vi "Main.vi"() -> ()   [LabVIEW 2013]
uses:
  <vilib>/Utility/miscctls.llb/LVPointDoubleTypeDef.ctl
  <vilib>/Analysis/1siggen.llb/Ramp Pattern by Samples.vi
  <vilib>/DAQmx/create/channels.llb/DAQmx Create Channel (AO-Voltage-Basic).vi
  <vilib>/Utility/file.llb/Write To Spreadsheet File (DBL).vi
  <vilib>/Analysis/NI_AALBase.lvlib
panel:
  out "Events A":i32
  out "Events B":i32
  in  "Tab Control":enum32{"Scan", "Correlations", "Setup"}(tab)
  in  "Init":bool
  in  "Release":bool
  in  "Save":bool
  in  "Goto Cursor":bool
  in  "Select":bool
  in  "Goto Zero":bool
  in  "Start Scan":bool
  out "Scanning":bool
  in  "dt (in tc)":u32
  out "Estimated Time (ms)":dbl
  in  "Dim1Scan":cluster{"Start":dbl, "Stop":dbl, "Steps":u32}={"Start"=0.0, "Stop"=0.0, "Steps"=1} {"Steps" min=1}
  in  "Dim1":u16(ring) items=["X", "Y", "Z"]
  in  "Dim2Scan":cluster{"Start":dbl, "Stop":dbl, "Steps":u32} {"Steps" min=1}
  in  "Dim2":u16(ring) items=["Y", "Z", "none"]
  in  "Dim3Scan":cluster{"Start":dbl, "Stop":dbl, "Steps":u32} {"Steps" min=1}
  in  "Dim3":u16(ring) items=["Z", "none"]
  out "XY Graph":T1(graph)
  out "Intensity Graph":dbl[][](graph)
  in  "3rd Dim":u32
  in  "2nd Dim":u32
  out "Cursor.Cursor Position":T2
  out "XY Graph 2":cluster{"Ramp Pattern":dbl[], "Data":i32[]}(graph)
  in  "Acquire":bool
  in  "Bin Size (ps)":i32
  in  "Bin Count":i32
  out "Voltage out":dbl[](array[numeric])
  in  "Relative Position":cluster{"X":dbl, "Y":dbl, "Z":dbl} {"Z" step=1.0; "Y" step=1.0; "X" step=1.0}
  in  "Voltage Step":cluster{"X":dbl, "Y":dbl, "Z":dbl}
  in  "Center Voltage":cluster{"X":dbl, "Y":dbl, "Z":dbl}
  in  "Define as center":bool
  out "Error":errorcluster
  in  "N":u32
  in  "Device ID":i32
  in  "Channel A":i32
  in  "Channel B":i32
  out "Time Base (ps)":dbl
  out "History Graph":cluster{dbl[], dbl[]}(graph)
  out "Value":dbl
  in  "tc (ms)":u32
  in  "stop":bool
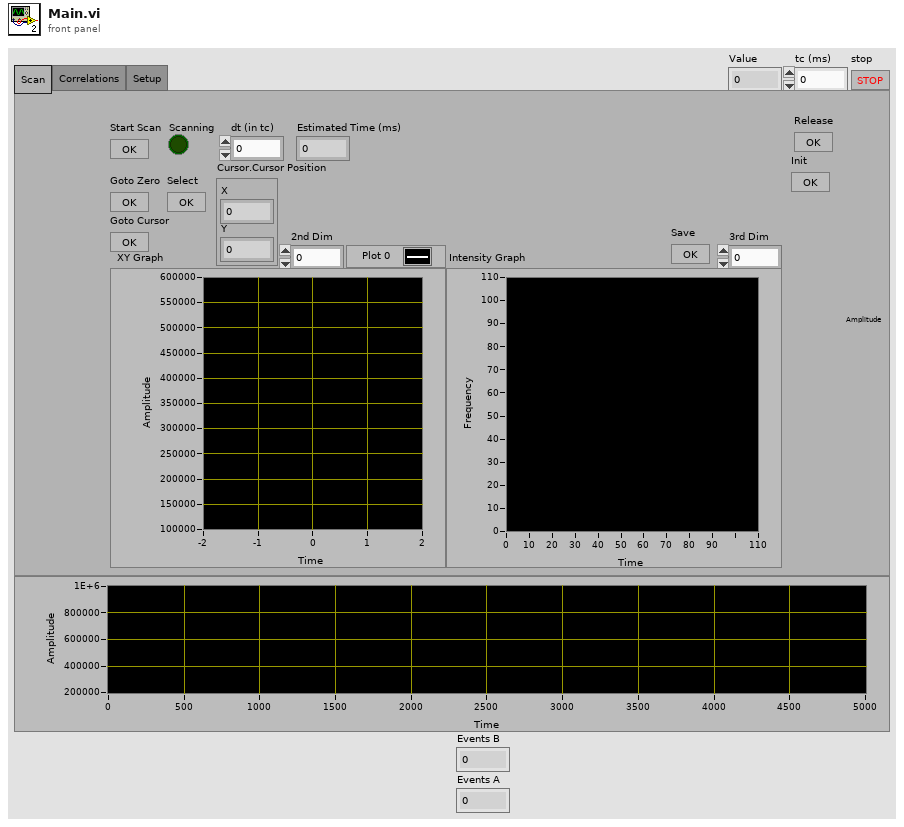
[diagram p1: front panel]
types:
  T1 = cluster{"Ramp Pattern":dbl[], "Ramp Pattern":dbl[]}
  T2 = typedef "LVPointDoubleTypeDef.ctl" = cluster{"X":dbl, "Y":dbl}
  T3 = cluster{"Voltage out[0]":dbl, "Voltage out[1]":dbl, "Voltage out[2]":dbl}
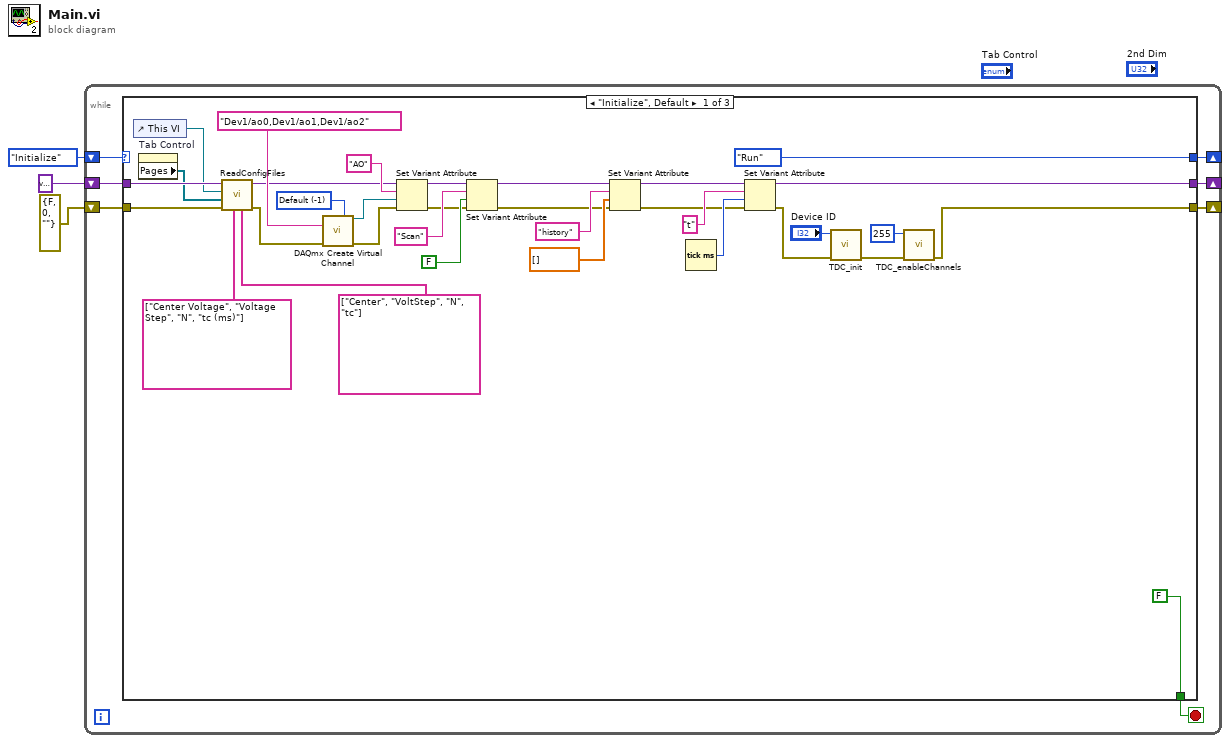
[diagram p0: block diagram]
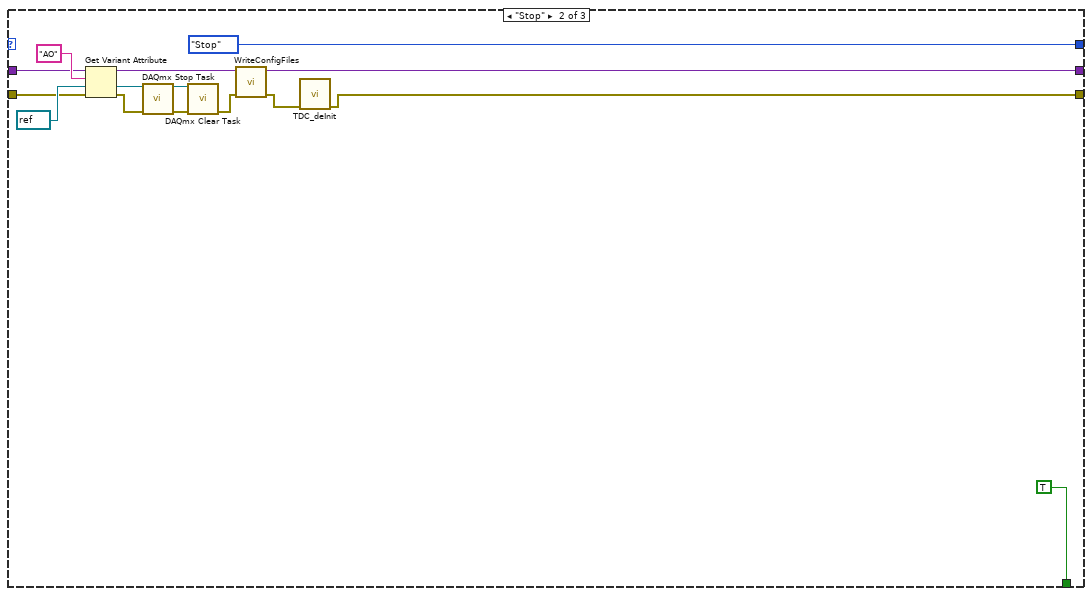
[diagram p2: hidden frame]
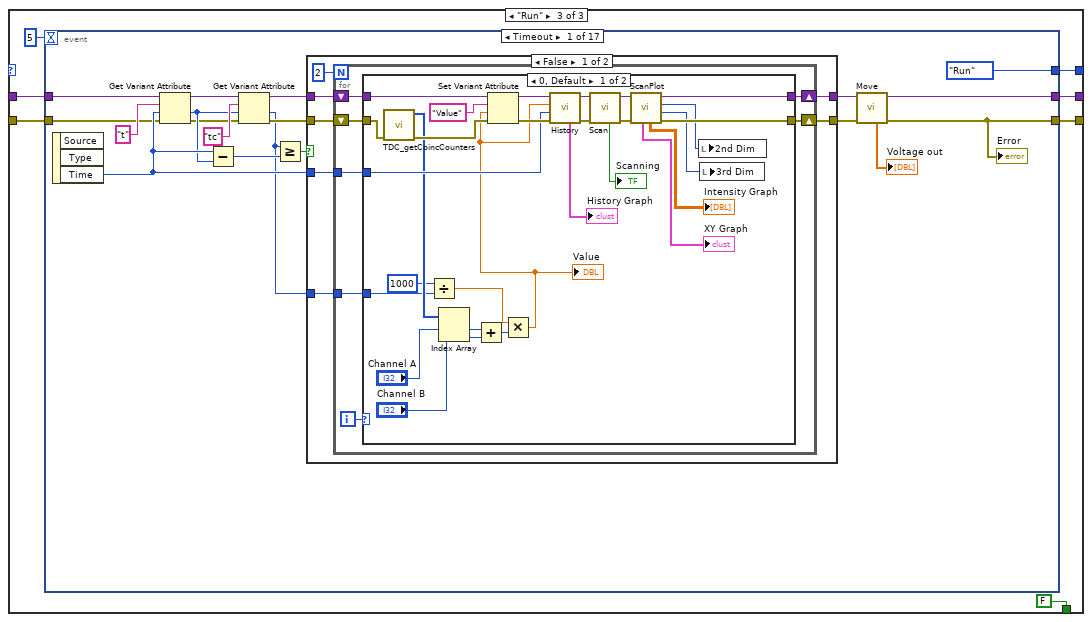
[diagram p3: hidden frame]
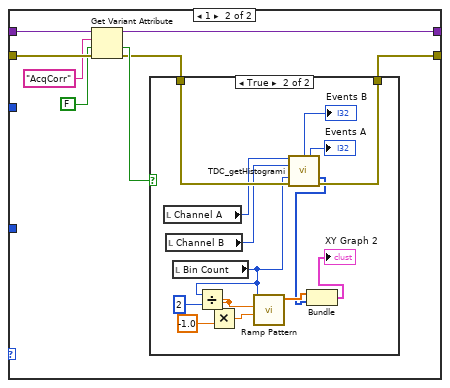
[diagram p4: hidden frame]
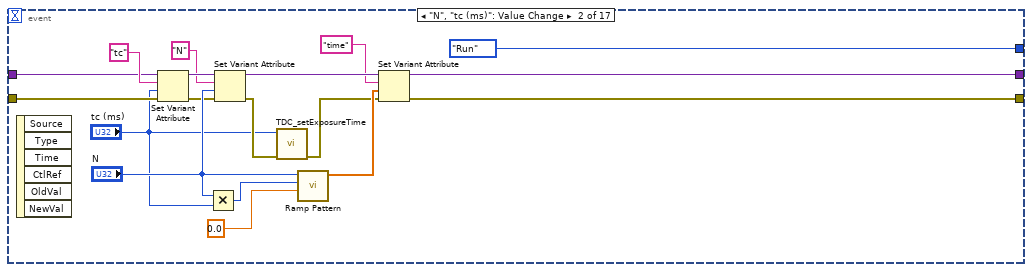
[diagram p7: hidden frame]
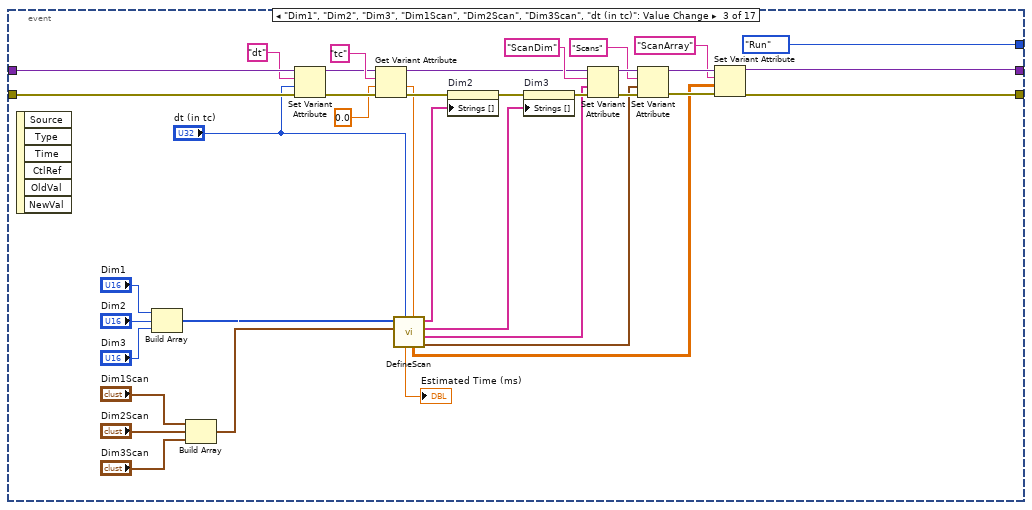
[diagram p8: hidden frame]
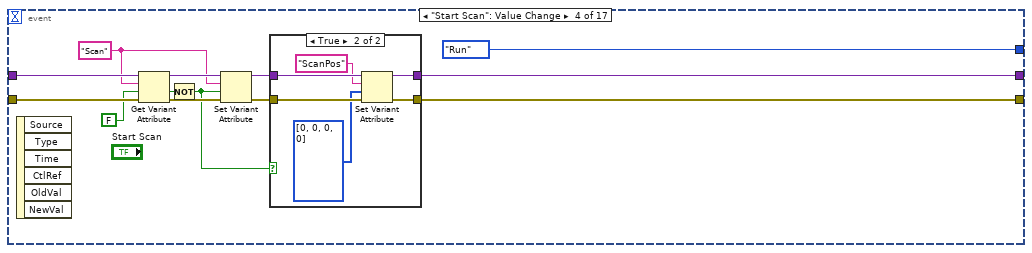
[diagram p9: hidden frame]
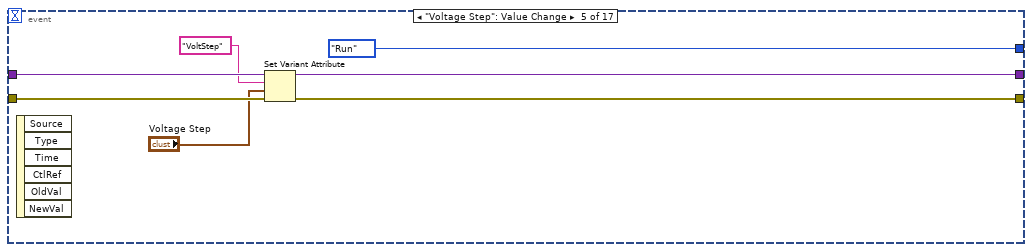
[diagram p11: hidden frame]
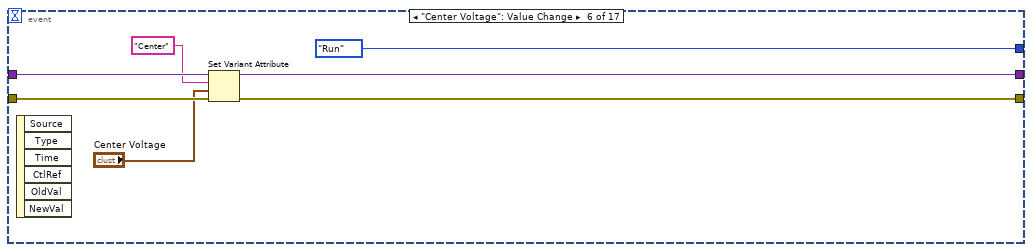
[diagram p12: hidden frame]
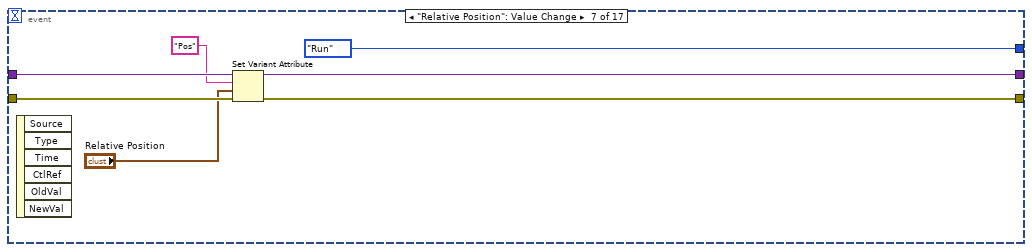
[diagram p13: hidden frame]
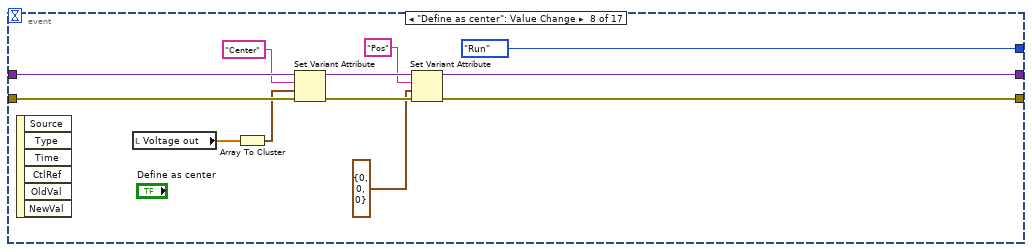
[diagram p14: hidden frame]
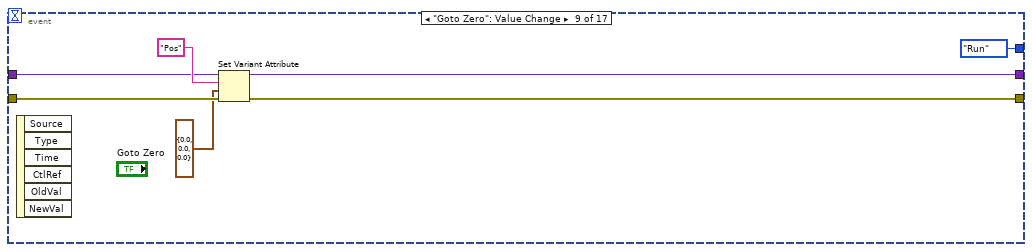
[diagram p15: hidden frame]
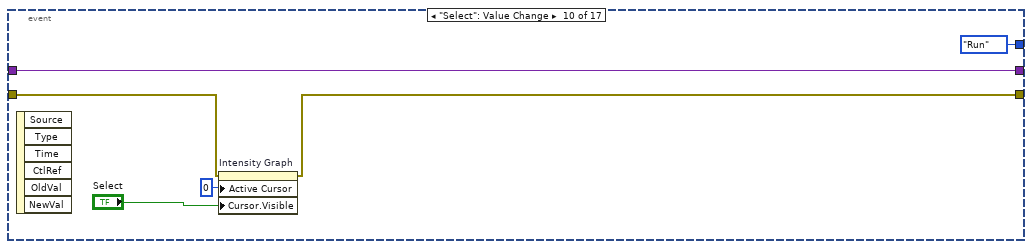
[diagram p16: hidden frame]
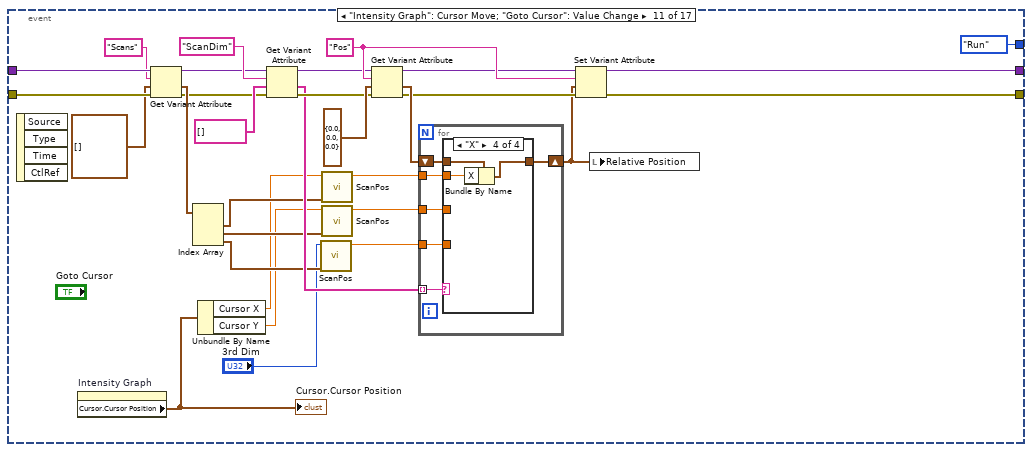
[diagram p17: hidden frame]
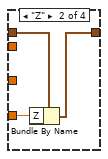
[diagram p19: hidden frame]
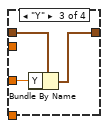
[diagram p20: hidden frame]
diagram:
  n1 = while {
    shift-right: [w9] -> _
    shift-left: enum16{"Initialize", "Run", "Stop"}."Initialize" -> [w10]
    shift-right: [w5] -> _
    shift-left: variant ("variant") -> [w7]
    shift-right: [w4] -> _
    shift-left: errorcluster {"status"=FALSE, "code"=0, "source"=""} ("error constant") -> [w6]
    stop <- w8 stop-if-true
    n2 = case shown="\"Initialize\", Default" w10 {
      tunnel: [enum16{"Initialize", "Run", "Stop"}."Run" enum16{"Initialize", "Run", "Stop"}."Stop" w65] -> w9
      tunnel: [FALSE TRUE FALSE] -> w8
      tunnel: w7 -> [w22 w54 w62]
      tunnel: w6 -> [w23 w53 w61]
      tunnel: [w35 w46 w60] -> w5
      tunnel: [w17 w44 w59] -> w4
      frame "Initialize", Default {
        w24 = -1 items=["Default"=-1, "RSE"=10083, "Differential"=10106, "Pseudodifferential"=12529] ("output terminal configuration")
        n3 = control-ref of="This VI"() -> (w14:refnum<vi>)
        n4 = property on="Tab Control" class="TabCtl (strict)"() -> ("Pages"=w13:refnum<vi>[])  [unwired: 2 in, 2 out]
        n5 = call "ReadConfigFiles.vi"("Variable"=string[] ["Center", "VoltStep", "N", "tc"], "Control"=string[] ["Center Voltage", "Voltage Step", "N", "tc (ms)"], "error in"=w23, "Pages"=w13, "reference"=w14, "variant in"=w22) -> ("error out"=w20:errorcluster, "variant out"=w21:variant)  [unwired: 4 in]
        n6 = call-poly <vilib>:"DAQmx Create Virtual Channel.vi"("output terminal configuration"=w24, "physical channels"=tag "Dev1/ao0,Dev1/ao1,Dev1/ao2", "error in"=w20) -> ("task out"=w28:refnum<k21>, "error out"=w29:errorcluster)  [unwired: 11 in]
        n7 = Set Variant Attribute(Variant=w21, name="AO", value=w28, error in=w29) -> (Variant out=w26:variant, error out=w25:errorcluster)  [unwired: 1 out]
        n8 = Set Variant Attribute(Variant=w26, name="Scan", value=FALSE, error in=w25) -> (Variant out=w34:variant, error out=w33:errorcluster)  [unwired: 1 out]
        n9 = Set Variant Attribute(Variant=w34, name="history", value=dbl[] [], error in=w33) -> (Variant out=w39:variant, error out=w36:errorcluster)  [unwired: 1 out]
        n10 = Tick Count (ms)() -> (millisecond timer value=w40:u32)
        n11 = Set Variant Attribute(Variant=w39, name="t", value=w40, error in=w36) -> (Variant out=w35:variant, error out=w19:errorcluster)  [unwired: 1 out]
        n12 = call "TDC_init.vi"("Error In"=w19, "Device ID"="Device ID") -> ("Error Out"=w18:errorcluster)  [unwired: 9 in]
        n13 = call "TDC_enableChannels.vi"("Error In"=w18, "channelMask"=255) -> ("Error Out"=w17:errorcluster)  [unwired: 9 in]
      }
      frame "Stop" {
        n14 = Get Variant Attribute(Variant=w54, name="AO", default value (empty Variant)=refnum<k21> refnum ("task out"), error in=w53) -> (duplicate Variant=w48:variant, value=w49:refnum<k21>, error out=w50:errorcluster)  [unwired: 1 out]
        n15 = call <vilib>:"DAQmx Stop Task.vi"("task/channels in"=w49, "error in"=w50) -> ("task out"=w52:refnum<k21>, "error out"=w51:errorcluster)  [unwired: 12 in]
        n16 = call <vilib>:"DAQmx Clear Task.vi"("task in"=w52, "error in"=w51) -> ("error out"=w47:errorcluster)  [unwired: 13 in]
        n17 = call "WriteConfigFiles.vi"("error in"=w47, "variant in"=w48) -> ("error out"=w45:errorcluster, "variant out"=w46:variant)  [unwired: 8 in]
        n18 = call "TDC_deInit.vi"("Error In"=w45) -> ("Error Out"=w44:errorcluster)  [unwired: 10 in]
      }
      frame "Run" {
        n19 = event shown="[0] Timeout" {
          selector: _ -> [_ _ _ _ _ _ _ _ _ _ _ _ _ _ _ _ _]
          dyn-events: _ -> [_ _ _ _ _ _ _ _ _ _ _ _ _ _ _ _ _]
          timeout: 5 -> [_ _ _ _ _ _ _ _ _ _ _ _ _ _ _ _ _]
          tunnel: [enum16{"Initialize", "Run", "Stop"}."Run" enum16{"Initialize", "Run", "Stop"}."Run" enum16{"Initialize", "Run", "Stop"}."Run" enum16{"Initialize", "Run", "Stop"}."Run" enum16{"Initialize", "Run", "Stop"}."Run" enum16{"Initialize", "Run", "Stop"}."Run" enum16{"Initialize", "Run", "Stop"}."Run" enum16{"Initialize", "Run", "Stop"}."Run" enum16{"Initialize", "Run", "Stop"}."Run" enum16{"Initialize", "Run", "Stop"}."Run" enum16{"Initialize", "Run", "Stop"}."Run" enum16{"Initialize", "Run", "Stop"}."Run" enum16{"Initialize", "Run", "Stop"}."Run" enum16{"Initialize", "Run", "Stop"}."Run" enum16{"Initialize", "Run", "Stop"}."Run" enum16{"Initialize", "Run", "Stop"}."Stop" enum16{"Initialize", "Run", "Stop"}."Stop"] -> w65
          tunnel: w62 -> [w73 w156 w202 w216 w231 w238 w245 w257 w263 w271 w301 w335 w348 w357 w370 w373 w380]
          tunnel: w61 -> [w72 w155 w201 w215 w230 w237 w244 w255 w262 w267 w300 w332 w347 w356 w369 w372 w377]
          tunnel: [w68 w154 w186 w206 w229 w236 w243 w254 w261 w271 w274 w335 w346 w355 w370 w373 w380] -> w60
          tunnel: [w67 w153 w185 w205 w228 w235 w242 w253 w260 w266 w273 w333 w342 w354 w369 w371 w376] -> w59
          event Timeout {
            n20 = event-data() -> ("Time"=w78:u32)  [unwired: 1 in, 2 out]
            n21 = Get Variant Attribute(Variant=w73, name="t", default value (empty Variant)=w78, error in=w72) -> (duplicate Variant=w77:variant, value=w75:u32, error out=w74:errorcluster)  [unwired: 1 out]
            n22 = Subtract(x=w78, y=w75) -> (x-y=w80:u32)
            n23 = Get Variant Attribute(Variant=w77, name="tc", default value (empty Variant)=w75, error in=w74) -> (duplicate Variant=w71:variant, value=w66:u32, error out=w70:errorcluster)  [unwired: 1 out]
            n24 = Greater Or Equal?(x=w66, y=w80) -> (x >= y?=w79:bool)
            n25 = case shown="False" w79 {
              tunnel: w78 -> [w88 _]
              tunnel: w71 -> [w89 w149]
              tunnel: w70 -> [w85 w148]
              tunnel: [w87 w149] -> w68
              tunnel: [w86 w148] -> w67
              tunnel: w66 -> [w84 _]
              frame False {
                n26 = for {
                  N: 2 -> [_]
                  tunnel: w88 -> [w95]
                  tunnel: w84 -> [w91]
                  shift-right: [w94] -> w87
                  shift-left: w89 -> [w96]
                  shift-right: [w93] -> w86
                  shift-left: w85 -> [w92]
                  i -> [w90]
                  n27 = case shown="0, Default" w90 {
                    tunnel: w96 -> [w124 w132]
                    tunnel: w95 -> [w119 _]
                    tunnel: [w114 w130] -> w94
                    tunnel: [w113 w125] -> w93
                    tunnel: w92 -> [w108 w131]
                    tunnel: w91 -> [w100 _]
                    frame 0, Default {
                      n28 = call "TDC_getCoincCounters.vi"("Error In"=w108) -> ("Error Out"=w107:errorcluster, "Coincidence Counters"=w106:i32[])  [unwired: 9 in]
                      n29 = Divide(x=1000, y=w100) -> (x/y=w98:dbl)
                      n30 = Index Array(array=w106, index #1="Channel A", index #2="Channel B") -> (element #1=w102:i32, element #2=w103:i32)
                      n31 = Add(x=w102, y=w103) -> (x+y=w99:i32)
                      n32 = Multiply(x=w98, y=w99) -> (x*y=w97:dbl)
                      "Value" <- w97
                      n33 = Set Variant Attribute(Variant=w124, name="Value", value=w97, error in=w107) -> (Variant out=w121:variant, error out=w122:errorcluster)  [unwired: 1 out]
                      n34 = call "History.vi"("error in"=w122, "time"=w119, "Value"=w97, "variant in"=w121) -> ("error out"=w117:errorcluster, "variant out"=w118:variant, "history graph"=→"History Graph":cluster{dbl[], dbl[]})  [unwired: 5 in]
                      n35 = call "Scan.vi"("error in"=w117, "variant in"=w118) -> ("error out"=w113:errorcluster, "variant out"=w115:variant, "Scanning"=→"Scanning":bool)  [unwired: 7 in]
                      n36 = call "ScanPlot.vi"("error in"=w113, "variant in"=w115) -> ("3rd Dim"=w111:u32, "2nd Dim"=w112:u32, "variant out"=w114:variant, "Intensity Graph"=→"Intensity Graph":dbl[][], "XY Graph"=→"XY Graph":T1)  [unwired: 4 in, 1 out]
                      n37 = local write "2nd Dim"(w112) -> ()
                      n38 = local write "3rd Dim"(w111) -> ()
                    }
                    frame 1 {
                      n39 = Get Variant Attribute(Variant=w132, name="AcqCorr", default value (empty Variant)=FALSE, error in=w131) -> (duplicate Variant=w130:variant, value=w127:bool, error out=w126:errorcluster)  [unwired: 1 out]
                      n40 = case shown="True" w127 {
                        tunnel: w126 -> [w133 w147]
                        tunnel: [w133 w146] -> w125
                        frame False {
                        }
                        frame True {
                          n41 = local read "Channel A"() -> (w145:i32)
                          n42 = local read "Channel B"() -> (w144:i32)
                          n43 = local read "Bin Count"() -> (w141:i32)
                          n44 = Divide(x=w141, y=2) -> (x/y=w138:dbl)
                          n45 = Multiply(x=w138, y=-1.0) -> (x*y=w139:dbl)
                          n46 = call-poly <vilib>:"Ramp Pattern.vi"("start"=w139, "end"=w138, "samples"=w141) -> ("Ramp Pattern"=w136:dbl[])  [unwired: 7 in, 1 out]
                          n47 = call "TDC_getHistogrami.vi"("Channel A"=w145, "Channel B"=w144, "Histogram Size"=w141, "Error In"=w147) -> ("Events B"=→"Events B":i32, "Events A"=→"Events A":i32, "Data"=w135:i32[], "Error Out"=w146:errorcluster)  [unwired: 4 in, 4 out]
                          n48 = Bundle("Ramp Pattern"=w136, "Data"=w135) -> (→"XY Graph 2":cluster{"Ramp Pattern":dbl[], "Data":i32[]})  [unwired: 1 in]
                        }
                      }
                    }
                  }
                }
              }
              frame True {
              }
            }
            "Error" <- w67
            n49 = call "Move.vi"("error in"=w67, "variant in"=w68) -> ("Voltage out"=→"Voltage out":dbl[])  [unwired: 7 in, 2 out]
          }
          event "N", "tc (ms)": Value Change {
            n50 = event-data() -> ()  [unwired: 1 in, 6 out]
            n51 = Set Variant Attribute(Variant=w156, name="tc", value="tc (ms)", error in=w155) -> (Variant out=w167:variant, error out=w157:errorcluster)  [unwired: 1 out]
            n52 = Multiply(x="N", y="tc (ms)") -> (x*y=w163:u32)
            n53 = Set Variant Attribute(Variant=w167, name="N", value="N", error in=w157) -> (Variant out=w161:variant, error out=w152:errorcluster)  [unwired: 1 out]
            n54 = call "TDC_setExposureTime.vi"("Error In"=w152, "Exposure Time [ms]"="tc (ms)") -> ("Error Out"=w151:errorcluster)  [unwired: 9 in]
            n55 = call-poly <vilib>:"Ramp Pattern.vi"("start"=0.0, "end"=w163, "samples"="N") -> ("Ramp Pattern"=w159:dbl[])  [unwired: 7 in, 1 out]
            n56 = Set Variant Attribute(Variant=w161, name="time", value=w159, error in=w151) -> (Variant out=w154:variant, error out=w153:errorcluster)  [unwired: 1 out]
          }
          event "Dim1", "Dim2", "Dim3", "Dim1Scan", "Dim2Scan", "Dim3Scan", "dt (in tc)": Value Change {
            n57 = event-data() -> ()  [unwired: 1 in, 6 out]
            n58 = Build Array("Dim1", "Dim2", "Dim3") -> (w175:u16[])
            n59 = Build Array("Dim1Scan", "Dim2Scan", "Dim3Scan") -> (w174:cluster{"Start":dbl, "Stop":dbl, "Steps":u32}[])
            n60 = Set Variant Attribute(Variant=w202, name="dt", value="dt (in tc)", error in=w201) -> (Variant out=w193:variant, error out=w192:errorcluster)  [unwired: 1 out]
            n61 = Get Variant Attribute(Variant=w193, name="tc", default value (empty Variant)=0.0, error in=w192) -> (duplicate Variant=w190:variant, value=w177:dbl, error out=w191:errorcluster)  [unwired: 1 out]
            n62 = call "DefineScan.vi"("tc"=w177, "dt (in tc)"="dt (in tc)", "DimensionScans"=w174, "Dimensions"=w175) -> ("Scans"=w168:cluster{"Start":dbl, "Stop":dbl, "Steps":u32}[], "ScanDim"=w169:string[], "Dim3Strings"=w170:string[], "Dim2Strings"=w171:string[], "ScanArray"=w172:dbl[][][], "Estimated Time (ms)"=→"Estimated Time (ms)":dbl)  [unwired: 2 in]
            n63 = property on="Dim2" class="Ring (strict)"(error in=w191, "Strings []"=w171) -> (error out=w203:errorcluster)  [unwired: 1 in, 1 out]
            n64 = property on="Dim3" class="Ring (strict)"(error in=w203, "Strings []"=w170) -> (error out=w198:errorcluster)  [unwired: 1 in, 1 out]
            n65 = Set Variant Attribute(Variant=w190, name="ScanDim", value=w169, error in=w198) -> (Variant out=w200:variant, error out=w199:errorcluster)  [unwired: 1 out]
            n66 = Set Variant Attribute(Variant=w200, name="Scans", value=w168, error in=w199) -> (Variant out=w188:variant, error out=w187:errorcluster)  [unwired: 1 out]
            n67 = Set Variant Attribute(Variant=w188, name="ScanArray", value=w172, error in=w187) -> (Variant out=w186:variant, error out=w185:errorcluster)  [unwired: 1 out]
          }
          event "Start Scan": Value Change {
            w212 = "Scan" ("name")
            n68 = event-data() -> ()  [unwired: 1 in, 6 out]
            n69 = Get Variant Attribute(Variant=w216, name=w212, default value (empty Variant)=FALSE, error in=w215) -> (duplicate Variant=w214:variant, value=w210:bool, error out=w213:errorcluster)  [unwired: 1 out]
            n70 = Not(x=w210) -> (.not. x?=w209:bool)
            n71 = Set Variant Attribute(Variant=w214, name=w212, value=w209, error in=w213) -> (Variant out=w208:variant, error out=w207:errorcluster)  [unwired: 1 out]
            n72 = case shown="True" w209 {
              tunnel: w208 -> [w219 w225]
              tunnel: w207 -> [w218 w224]
              tunnel: [w219 w221] -> w206
              tunnel: [w218 w220] -> w205
              frame False {
              }
              frame True {
                n73 = Set Variant Attribute(Variant=w225, name="ScanPos", value=i32[] [0, 0, 0, 0], error in=w224) -> (Variant out=w221:variant, error out=w220:errorcluster)  [unwired: 1 out]
              }
            }
          }
          event "Voltage Step": Value Change {
            n74 = event-data() -> ()  [unwired: 1 in, 6 out]
            n75 = Set Variant Attribute(Variant=w231, name="VoltStep", value="Voltage Step", error in=w230) -> (Variant out=w229:variant, error out=w228:errorcluster)  [unwired: 1 out]
          }
          event "Center Voltage": Value Change {
            n76 = event-data() -> ()  [unwired: 1 in, 6 out]
            n77 = Set Variant Attribute(Variant=w238, name="Center", value="Center Voltage", error in=w237) -> (Variant out=w236:variant, error out=w235:errorcluster)  [unwired: 1 out]
          }
          event "Relative Position": Value Change {
            n78 = event-data() -> ()  [unwired: 1 in, 6 out]
            n79 = Set Variant Attribute(Variant=w245, name="Pos", value="Relative Position", error in=w244) -> (Variant out=w243:variant, error out=w242:errorcluster)  [unwired: 1 out]
          }
          event "Define as center": Value Change {
            n80 = event-data() -> ()  [unwired: 1 in, 6 out]
            n81 = local read "Voltage out"() -> (w251:dbl[])
            n82 = Array To Cluster(array=w251) -> (cluster=w250:T3)
            n83 = Set Variant Attribute(Variant=w257, name="Center", value=w250, error in=w255) -> (Variant out=w256:variant, error out=w252:errorcluster)  [unwired: 1 out]
            n84 = Set Variant Attribute(Variant=w256, name="Pos", value=cluster{"X":i32, "Y":i32, "Z":i32} {"X"=0, "Y"=0, "Z"=0} ("Relative Position"), error in=w252) -> (Variant out=w254:variant, error out=w253:errorcluster)  [unwired: 1 out]
          }
          event "Goto Zero": Value Change {
            n85 = event-data() -> ()  [unwired: 1 in, 6 out]
            n86 = Set Variant Attribute(Variant=w263, name="Pos", value=cluster{"X":dbl, "Y":dbl, "Z":dbl} {"X"=0.0, "Y"=0.0, "Z"=0.0} ("Relative Position"), error in=w262) -> (Variant out=w261:variant, error out=w260:errorcluster)  [unwired: 1 out]
          }
          event "Select": Value Change {
            n87 = event-data() -> ()  [unwired: 1 in, 6 out]
            n88 = property on="Intensity Graph" class="IntGraph (strict)"(error in=w267, "Active Cursor"=u32 0, "Cursor.Visible"="Select") -> (error out=w266:errorcluster)  [unwired: 1 in, 1 out]
          }
          event "Intensity Graph": Cursor Move; "Goto Cursor": Value Change {
            w291 = "Pos" ("name")
            n89 = event-data() -> ()  [unwired: 1 in, 4 out]
            n90 = property on="Intensity Graph" class="IntGraph (strict)"() -> ("Cursor.Cursor Position"=w278:T2)  [unwired: 2 in, 2 out]
            "Cursor.Cursor Position" <- w278
            n91 = Get Variant Attribute(Variant=w301, name="Scans", default value (empty Variant)=cluster{"Start":dbl, "Stop":dbl, "Steps":u32}[] [], error in=w300) -> (duplicate Variant=w286:variant, value=w297:cluster{"Start":dbl, "Stop":dbl, "Steps":u32}[], error out=w285:errorcluster)  [unwired: 1 out]
            n92 = Index Array(array=w297) -> (element #1=w281:cluster{"Start":dbl, "Stop":dbl, "Steps":u32}, element #2=w280:cluster{"Start":dbl, "Stop":dbl, "Steps":u32}, element #3=w279:cluster{"Start":dbl, "Stop":dbl, "Steps":u32})  [unwired: 3 in]
            n93 = Unbundle By Name(w278) -> ("Cursor X"=w277:dbl, "Cursor Y"=w276:dbl)
            n94 = Get Variant Attribute(Variant=w286, name="ScanDim", default value (empty Variant)=string[] [], error in=w285) -> (duplicate Variant=w284:variant, value=w282:string[], error out=w283:errorcluster)  [unwired: 1 out]
            n95 = call "ScanPos.vi"("DimScan"=w279, "ScanPos"="3rd Dim") -> ("Pos"=w295:dbl)  [unwired: 9 in]
            n96 = call "ScanPos.vi"("DimScan"=w281, "ScanPos"=w277) -> ("Pos"=w294:dbl)  [unwired: 9 in]
            n97 = call "ScanPos.vi"("DimScan"=w280, "ScanPos"=w276) -> ("Pos"=w296:dbl)  [unwired: 9 in]
            n98 = Get Variant Attribute(Variant=w284, name=w291, default value (empty Variant)=cluster{"X":dbl, "Y":dbl, "Z":dbl} {"X"=0.0, "Y"=0.0, "Z"=0.0} ("Relative Position"), error in=w283) -> (duplicate Variant=w289:variant, value=w292:cluster{"X":dbl, "Y":dbl, "Z":dbl}, error out=w290:errorcluster)  [unwired: 1 out]
            n99 = for {
              tunnel: w282 -> [w308] mode=indexing
              shift-right: [w306] -> w272
              shift-left: w292 -> [w307]
              tunnel: w294 -> [w305]
              tunnel: w295 -> [w304]
              tunnel: w296 -> [w303]
              n100 = case shown="\"X\"" w308 {
                tunnel: w307 -> [w309 w312 w315 w318]
                tunnel: [w309 w311 w314 w317] -> w306
                tunnel: w305 -> [_ _ _ w316]
                tunnel: w304 -> [_ w310 _ _]
                tunnel: w303 -> [_ _ w313 _]
                frame "none", Default {
                }
                frame "Z" {
                  n101 = Bundle By Name(cluster=w312, "Z"=w310) -> (w311:cluster{"X":dbl, "Y":dbl, "Z":dbl})
                }
                frame "Y" {
                  n102 = Bundle By Name(cluster=w315, "Y"=w313) -> (w314:cluster{"X":dbl, "Y":dbl, "Z":dbl})
                }
                frame "X" {
                  n103 = Bundle By Name(cluster=w318, "X"=w316) -> (w317:cluster{"X":dbl, "Y":dbl, "Z":dbl})
                }
              }
            }
            n104 = Set Variant Attribute(Variant=w289, name=w291, value=w272, error in=w290) -> (Variant out=w274:variant, error out=w273:errorcluster)  [unwired: 1 out]
            n105 = local write "Relative Position"(w272) -> ()
          }
          event "Bin Count", "Bin Size (ps)": Value Change {
            w323 = 2 ("y")
            w324 = 2 ("y")
            n106 = event-data() -> ()  [unwired: 1 in, 6 out]
            n107 = call "TDC_getTimebase.vi"() -> ("Time Base [s]"=w331:dbl)  [unwired: 11 in]
            n108 = Multiply(x=w331, y=1000000000000.0) -> (x*y=w319:dbl)
            "Time Base (ps)" <- w319
            n109 = Divide(x="Bin Size (ps)", y=w319) -> (x/y=w326:dbl)
            n110 = Round To Nearest(number=w326) -> (nearest integer value=w325:dbl)
            n111 = Greater?(x=w325, y=w324) -> (0:w328:bool)
            n112 = case shown="False" w328 {
              tunnel: [w340 w341] -> w327
              tunnel: w325 -> [_ w341]
              tunnel: w324 -> [w340 _]
              tunnel: w319 -> [w339 _]
              frame False {
                n113 = Multiply(x=w340, y=w339) -> (x*y=w338:dbl)
                n114 = local write "Bin Size (ps)"(w338) -> ()
              }
              frame True {
              }
            }
            n115 = Greater?(x="Bin Count", y=w323) -> (0:w322:bool)
            n116 = case shown="False" w322 {
              tunnel: [w336 w337] -> w320
              tunnel: "Bin Count" -> [_ w337]
              tunnel: w323 -> [w336 _]
              frame False {
                n117 = local write "Bin Count"(w336) -> ()
              }
              frame True {
              }
            }
            n118 = call "TDC_setHistogramParams.vi"("Error In"=w332, "Bin Count"=w320, "Bin Width [native bins]"=w327) -> ("Error Out"=w333:errorcluster)  [unwired: 8 in]
          }
          event "Acquire": Value Change {
            n119 = event-data() -> ()  [unwired: 1 in, 6 out]
            n120 = Set Variant Attribute(Variant=w348, name="AcqCorr", value="Acquire", error in=w347) -> (Variant out=w346:variant, error out=w343:errorcluster)  [unwired: 1 out]
            n121 = case shown="False" "Acquire" {
              tunnel: w343 -> [w350 w352]
              tunnel: [w350 w351] -> w342
              frame False {
              }
              frame True {
                n122 = call "TDC_clearAllHistograms.vi"("Error In"=w352) -> ("Error Out"=w351:errorcluster)  [unwired: 10 in]
              }
            }
          }
          event "Save": Value Change {
            n123 = event-data() -> ()  [unwired: 1 in, 6 out]
            n124 = Get Variant Attribute(Variant=w357, name="ScanPos", default value (empty Variant)=i32[] [0, 0, 0, 0], error in=w356) -> (duplicate Variant=w362:variant, value=w363:i32[], error out=w361:errorcluster)  [unwired: 1 out]
            n125 = Index Array(array=w363) -> (element #4=w366:i32)  [unwired: 4 in, 3 out]
            n126 = Get Variant Attribute(Variant=w362, name="ScanArray", default value (empty Variant)=dbl[][][] [] ("initialized array"), error in=w361) -> (duplicate Variant=w355:variant, value=w358:dbl[][][], error out=w354:errorcluster)  [unwired: 1 out]
            n127 = Index Array(array=w358, index (dim 2)=w366) -> (element=w353:dbl[][])  [unwired: 2 in]
            n128 = call-poly <vilib>:"Write To Spreadsheet File.vi"("2D data"=w353) -> ()  [unwired: 7 in, 1 out]
          }
          event "Release": Value Change {
            n129 = event-data() -> ()  [unwired: 1 in, 6 out]
          }
          event "stop": Value Change {
            n130 = event-data() -> ()  [unwired: 1 in, 6 out]
            n131 = call "TDC_deInit.vi"("Error In"=w372) -> ("Error Out"=w371:errorcluster)  [unwired: 10 in]
          }
          event "Init": Value Change {
            n132 = event-data() -> ()  [unwired: 1 in, 6 out]
            n133 = local read "Device ID"() -> (w375:i32)
            n134 = call "TDC_init.vi"("Error In"=w377, "Device ID"=w375) -> ("Error Out"=w379:errorcluster)  [unwired: 9 in]
            n135 = call "TDC_enableChannels.vi"("Error In"=w379, "channelMask"=255) -> ("Error Out"=w376:errorcluster)  [unwired: 9 in]
          }
        }
      }
    }
  }
